vi "Query Non-Linearity Correction Coefficient.vi"(8 "error in (no error)":errorcluster, 11 "VISA resource name":refnum<visa-resource-name>) -> (0 "error out":errorcluster, 1 "Non-Linearity Correction Order":dbl, 2 "Non-Linearity Correction Coefficient":dbl[](array[numeric]), 3 "VISA resource name out":refnum<visa-resource-name>)   [LabVIEW 2019, in "Ocean Optics 2000 4000.lvlib"]
doc: "Returns the non-linearity correction coefficients and also the correction order. These information are stored in the EEPROM.\n\nThe non-linearity correction coefficients define a polynomial and used to compute a scaling factor. This correction is intended for overcoming some nonlinearity in the response of the sensor to light with respect to integration time."
uses:
  Ocean Optics 2000 4000.lvlib
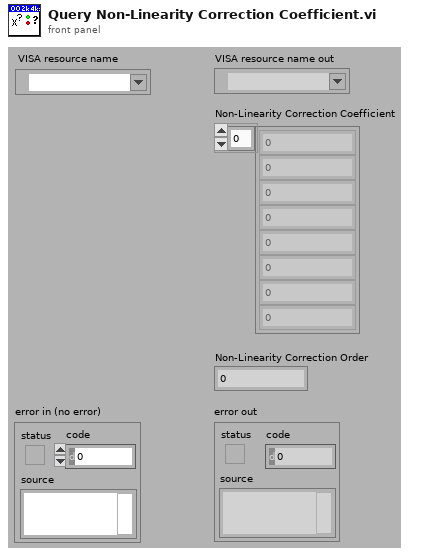
[diagram p1: front panel]
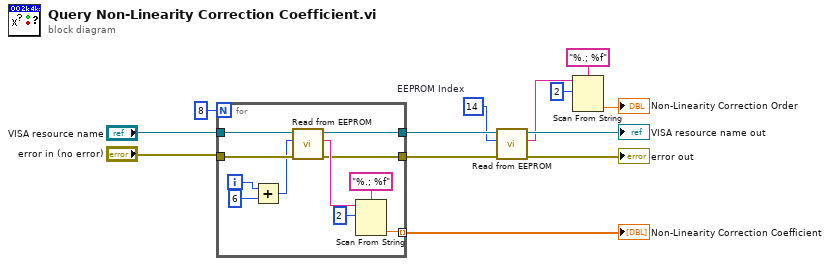
[diagram p0: block diagram]
diagram:
  w6 = u8 14  # EEPROM Index
  n1 = for {
    N: 8 -> [_]
    tunnel: "VISA resource name" -> [w24]
    tunnel: "error in (no error)" -> [w23]
    tunnel: [w17] -> w10 mode=indexing
    tunnel: [w15] -> w8
    tunnel: [w14] -> w7
    i -> [w21]
    n2 = Add(x=w21, y=6) -> (x+y=w22:i32)
    n3 = call "Read from EEPROM.vi"("error in (no error)"=w23, "EEPROM Index"=w22, "VISA resource name"=w24) -> ("error out"=w14:errorcluster, "ASCII Data"=w19:string, "VISA resource name out"=w15:refnum<visa-resource-name>)  [unwired: 6 out]
    n4 = Scan From String(format string="%.; %f", input string=w19, initial scan location=u32 2) -> (output 1=w17:dbl)  [unwired: 1 in, 4 out]
  }
  "Non-Linearity Correction Coefficient" <- w10
  n5 = call "Read from EEPROM.vi"("error in (no error)"=w7, "EEPROM Index"=w6, "VISA resource name"=w8) -> ("error out"=→"error out":errorcluster, "ASCII Data"=w2:string, "VISA resource name out"=→"VISA resource name out":refnum<visa-resource-name>)  [unwired: 6 out]
  n6 = Scan From String(format string="%.; %f", input string=w2, initial scan location=u32 2) -> (output 1=→"Non-Linearity Correction Order":dbl)  [unwired: 1 in, 4 out]
